vi "Populate_Do.vi"(8 "error in (no error)":errorcluster, 9 "Value":string, 10 "Lower case name":string, 11 "Caraya Unit Test in":refnum<class "Caraya Unit Test.lvclass">) -> (0 "error out":errorcluster, 1 "Success?":bool, 3 "Caraya Unit Test out":refnum<class "Caraya Unit Test.lvclass">)   [LabVIEW 2020, in "ProjectBuilder.lvlib" / "Caraya Unit Test.lvclass"]
uses:
  Caraya Unit Test.lvclass
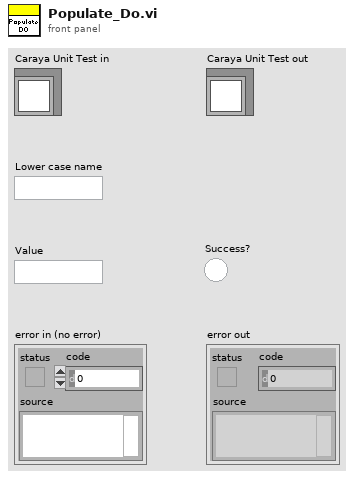
[diagram p1: front panel]
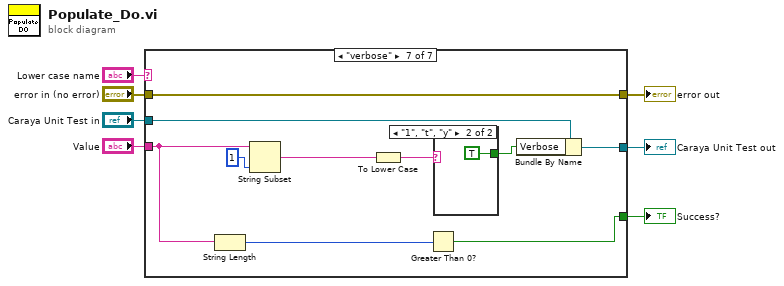
[diagram p0: block diagram]
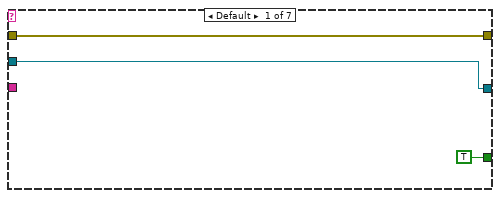
[diagram p2: hidden frame]
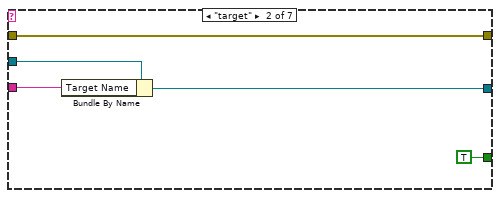
[diagram p3: hidden frame]
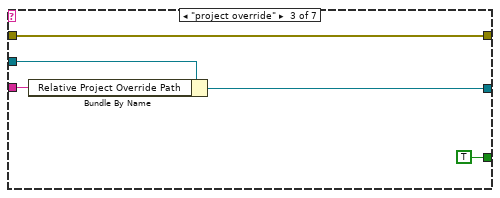
[diagram p4: hidden frame]
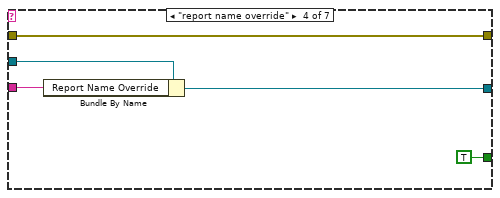
[diagram p5: hidden frame]
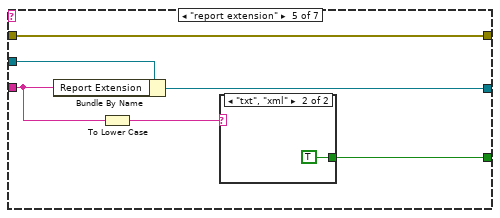
[diagram p6: hidden frame]
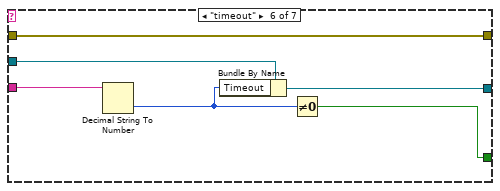
[diagram p8: hidden frame]
diagram:
  n1 = case shown="\"verbose\"" "Lower case name" {
    tunnel: [TRUE TRUE TRUE TRUE w26 w34 w39] -> w3
    tunnel: [w9 w14 w19 w24 w30 w37 w47] -> w2
    tunnel: "Caraya Unit Test in" -> [w9 w15 w20 w25 w31 w38 w48]
    tunnel: [w8 w12 w17 w22 w29 w36 w46] -> w1
    tunnel: "error in (no error)" -> [w8 w12 w17 w22 w29 w36 w46]
    tunnel: "Value" -> [_ w13 w18 w23 w28 w35 w41]
    frame Default {
    }
    frame "target" {
      n2 = Bundle By Name(cluster=w15, "Target Name"=w13) -> (w14:refnum<class "Caraya Unit Test.lvclass">)
    }
    frame "project override" {
      n3 = Bundle By Name(cluster=w20, "Relative Project Override Path"=w18) -> (w19:refnum<class "Caraya Unit Test.lvclass">)
    }
    frame "report name override" {
      n4 = Bundle By Name(cluster=w25, "Report Name Override"=w23) -> (w24:refnum<class "Caraya Unit Test.lvclass">)
    }
    frame "report extension" {
      n5 = Bundle By Name(cluster=w31, "Report Extension"=w28) -> (w30:refnum<class "Caraya Unit Test.lvclass">)
      n6 = To Lower Case(string=w28) -> (all lower case string=w27:string)
      n7 = case shown="\"txt\", \"xml\"" w27 {
        tunnel: [_ TRUE] -> w26
        frame Default {
        }
        frame "txt", "xml" {
        }
      }
    }
    frame "timeout" {
      n8 = Decimal String To Number(string=w35) -> (number=w33:i32)  [unwired: 2 in, 1 out]
      n9 = Bundle By Name(cluster=w38, "Timeout"=w33) -> (w37:refnum<class "Caraya Unit Test.lvclass">)
      n10 = Not Equal To 0?(x=w33) -> (x != 0?=w34:bool)
    }
    frame "verbose" {
      n11 = String Length(string=w41) -> (length=w40:i32)
      n12 = String Subset(string=w41, length (rest)=1 ("length (rest)")) -> (substring=w44:string)  [unwired: 1 in]
      n13 = To Lower Case(string=w44) -> (all lower case string=w43:string)
      n14 = Greater Than 0?(x=w40) -> (x > 0?=w39:bool)
      n15 = case shown="\"1\", \"t\", \"y\"" w43 {
        tunnel: [_ TRUE] -> w42
        frame Default {
        }
        frame "1", "t", "y" {
        }
      }
      n16 = Bundle By Name(cluster=w48, "Verbose"=w42) -> (w47:refnum<class "Caraya Unit Test.lvclass">)
    }
  }
  "error out" <- w1
  "Caraya Unit Test out" <- w2
  "Success?" <- w3
